vi "Apply Filter.vi"   [LabVIEW 2013, in "CVT editor node.lvclass"]
uses:
  CVT editor node.lvclass
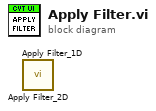
[diagram p0: block diagram]
diagram:
  n1 = call "Apply Filter_2D.vi"() -> ()  [unwired: 11 in, 1 out]
  n2 = call "Apply Filter_1D.vi"() -> ()  [unwired: 11 in, 1 out]
